vi "OneBallAuton.vi"   [LabVIEW 2013]
uses:
  <vilib>/Rock Robotics/WPI/SafetyOutput/WPI_SafetyOutputConfigMenu.ctl
  <vilib>/Rock Robotics/WPI/Solenoid/WPI_SolenoidValue.ctl
  <vilib>/Rock Robotics/WPI/RobotDrive/WPI_RobotDriveGetSetRefNum.vi
  <vilib>/Rock Robotics/WPI/Solenoid/WPI_SolenoidSetEnum.vi
types:
  T1 = typedef "WPI_SafetyOutputConfigMenu.ctl" = enum16{"Enable", "Disable"}
  T2 = typedef "WPI_RobotDriveDevRef.ctl" = cluster{"DevStatus":errorcluster, "Motors[]":T3[], "Square Inputs":bool, "Max Output":dbl, "Isochronous":bool}
  T3 = typedef "WPI_MotorControlDeviceRef.ctl" = cluster{"DeviceStatus":errorcluster, "Type":enum16{"PWM", "CAN"}, "PWM":cluster{"Digital Module":T4, "PWM Channel":T5, "DeadBand":T6}, "CAN":cluster{"Device Number":u8, "Control Mode":T7, "Semaphore":T8, "Max Vout":dbl}, "Invert":bool, "TransformRef":T9, "InvTransformRef":T9}
  T4 = typedef "FPGA_TypedefDigitalModule.ctl" = enum16{"Digital Module 1", "Digital Module 2"}
  T5 = typedef "FPGA_DIOPWMChannel.ctl" = enum8{"PWM 1", "PWM 2", "PWM 3", "PWM 4", "PWM 5", "PWM 6", "PWM 7", "PWM 8", "PWM 9", "PWM 10", "Invalid"}
  T6 = typedef "WPI_PWMDeadband.ctl" = cluster{"Name":string, "maxPositivePwm":i32, "minPositivePwm":i32, "centerPwm":i32, "maxNegativePwm":i32, "minNegativePwm":i32, "angularRange":u16}
  T7 = typedef "WPI_CANJaguar_ControlMode.ctl" = enum8{"Percent VBus", "Current", "Speed", "Position", "Voltage"}
  T8 = typedef "Semaphore RefNum" = refnum<k1>
  T9 = typedef "WPI_PWMTransform_ConPane.ctl" = refnum<vi>
  T10 = typedef "WPI_SolenoidDevRef.ctl" = cluster{"DevStatus":errorcluster, "Solenoid Module":T11, "Forward Solenoid Channel":T12, "Reverse Solenoid Channel":T12}
  T11 = typedef "FPGA_TypedefSolenoidModule.ctl" = enum16{"Solenoid Module 1", "Solenoid Module 2"}
  T12 = typedef "WPI_SolenoidChannel.ctl" = enum8{"Solenoid 1", "Solenoid 2", "Solenoid 3", "Solenoid 4", "Solenoid 5", "Solenoid 6", "Solenoid 7", "Solenoid 8", "Invalid"}
  T13 = typedef "WPI_DigitalInputDevRef.ctl" = cluster{"DevStatus":errorcluster, "DIO Channel":T14, "Digital Module":T4}
  T14 = typedef "FPGA_DIOChannel.ctl" = enum8{"DIO 1", "DIO 2", "DIO 3", "DIO 4", "DIO 5", "DIO 6", "DIO 7", "DIO 8", "DIO 9", "DIO 10", "DIO 11", "DIO 12", "DIO 13", "DIO 14", "Invalid"}
  T15 = typedef "WPI_EncoderDevRef.ctl" = cluster{"DevStatus":errorcluster, "EncoderIndex":T16, "CounterIndex":T17, "DistancePerCount":dbl, "Decoding Type":T18}
  T16 = typedef "FPGA_EncoderIdx.ctl" = enum8{"Enc 0", "Enc 1", "Enc 2", "Enc 3", "Invalid"}
  T17 = typedef "FPGA_CounterCtrSystemIndex.ctl" = enum8{"Ctr 0", "Ctr 1", "Ctr 2", "Ctr 3", "Ctr 4", "Ctr 5", "Ctr 6", "Ctr 7", "Invalid"}
  T18 = typedef "WPI_EncoderType.ctl" = enum16{"1x", "2x", "4x"}
  T19 = typedef "WPI_SolenoidValue.ctl" = enum16{"Off", "On", "Forward", "Reverse"}
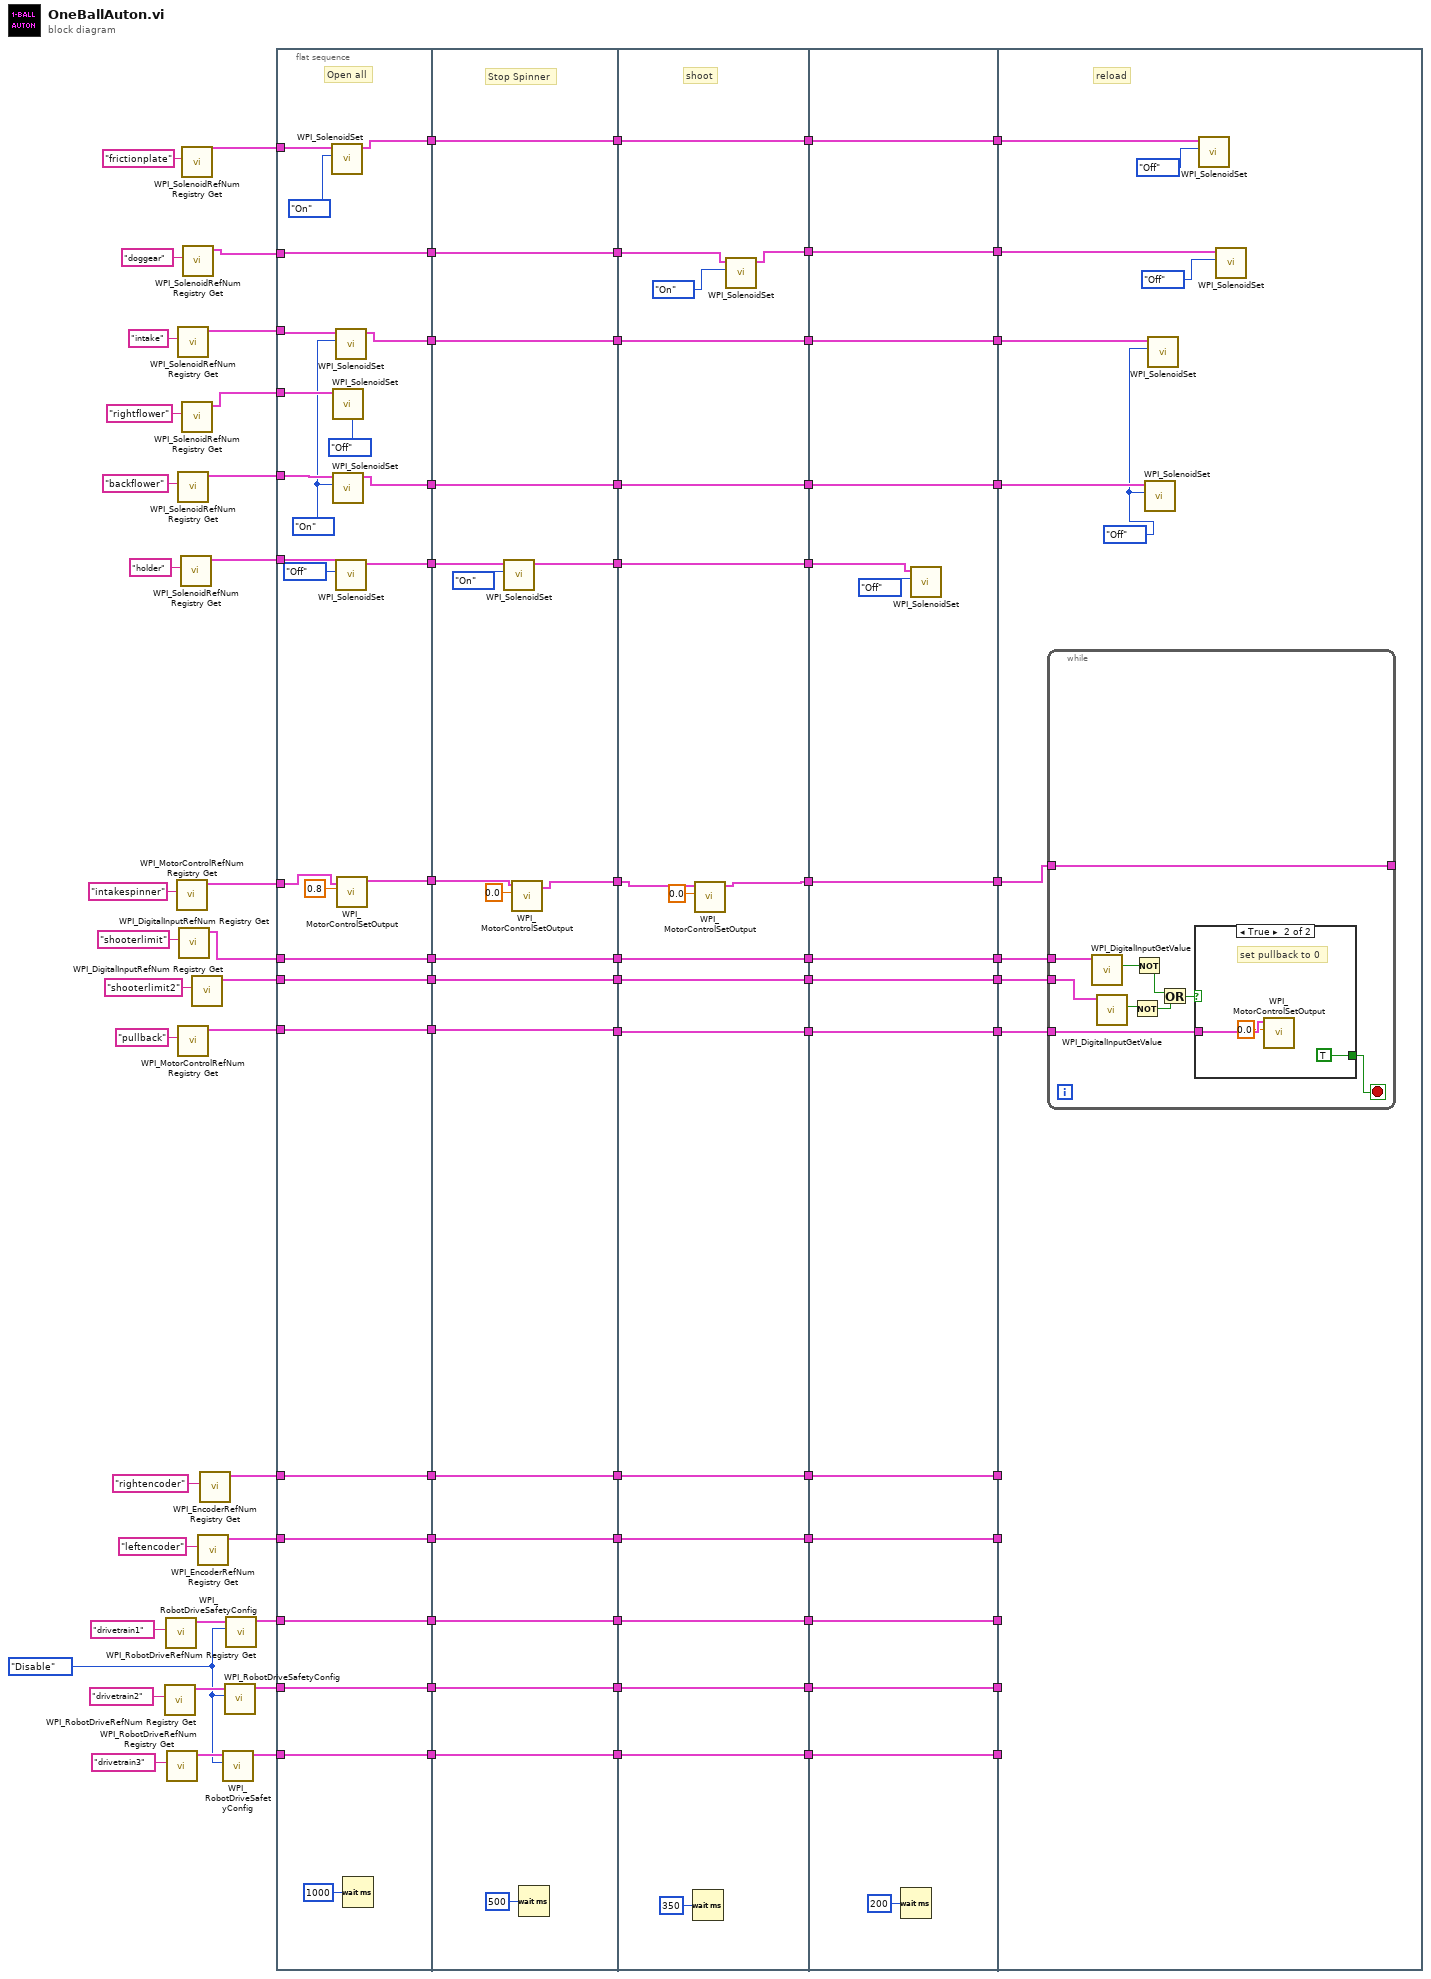
[diagram p0: block diagram]
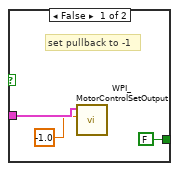
[diagram p2: hidden frame]
diagram:
  w49 = WPI_SafetyOutputConfigMenu."Disable" ("mode")
  n1 = call <vilib>:"WPI_RobotDriveRefNum Registry Get.vi"("refnum name"="drivetrain2") -> ("RobotDriveDevRef"=w51:T2)  [unwired: 9 in, 1 out]
  n2 = call <vilib>:"WPI_RobotDriveRefNum Registry Get.vi"("refnum name"="drivetrain1") -> ("RobotDriveDevRef"=w52:T2)  [unwired: 9 in, 1 out]
  n3 = call <vilib>:"WPI_RobotDriveRefNum Registry Get.vi"("refnum name"="drivetrain3") -> ("RobotDriveDevRef"=w50:T2)  [unwired: 9 in, 1 out]
  n4 = call <vilib>:"WPI_MotorControlRefNum Registry Get.vi"("refnum name"="intakespinner") -> ("MotorControlDevRef"=w62:T3)  [unwired: 9 in, 1 out]
  n5 = call <vilib>:"WPI_SolenoidRefNum Registry Get.vi"("refnum name"="intake") -> ("SolenoidDevRef"=w66:T10)  [unwired: 9 in, 1 out]
  n6 = call <vilib>:"WPI_SolenoidRefNum Registry Get.vi"("refnum name"="backflower") -> ("SolenoidDevRef"=w64:T10)  [unwired: 9 in, 1 out]
  n7 = call <vilib>:"WPI_MotorControlRefNum Registry Get.vi"("refnum name"="pullback") -> ("MotorControlDevRef"=w58:T3)  [unwired: 9 in, 1 out]
  n8 = call <vilib>:"WPI_DigitalInputRefNum Registry Get.vi"("refnum name"="shooterlimit") -> ("DigitalInputDevRef"=w60:T13)  [unwired: 9 in, 1 out]
  n9 = call <vilib>:"WPI_SolenoidRefNum Registry Get.vi"("refnum name"="holder") -> ("SolenoidDevRef"=w30:T10)  [unwired: 9 in, 1 out]
  n10 = call <vilib>:"WPI_SolenoidRefNum Registry Get.vi"("refnum name"="frictionplate") -> ("SolenoidDevRef"=w42:T10)  [unwired: 9 in, 1 out]
  n11 = call <vilib>:"WPI_SolenoidRefNum Registry Get.vi"("refnum name"="rightflower") -> ("SolenoidDevRef"=w65:T10)  [unwired: 9 in, 1 out]
  n12 = call <vilib>:"WPI_SolenoidRefNum Registry Get.vi"("refnum name"="doggear") -> ("SolenoidDevRef"=w70:T10)  [unwired: 9 in, 1 out]
  n13 = call <vilib>:"WPI_DigitalInputRefNum Registry Get.vi"("refnum name"="shooterlimit2") -> ("DigitalInputDevRef"=w34:T13)  [unwired: 9 in, 1 out]
  n14 = call <vilib>:"WPI_EncoderRefNum Registry Get.vi"("refnum name"="leftencoder") -> ("EncoderDevRef"=w47:T15)  [unwired: 9 in, 1 out]
  n15 = call <vilib>:"WPI_EncoderRefNum Registry Get.vi"("refnum name"="rightencoder") -> ("EncoderDevRef"=w48:T15)  [unwired: 9 in, 1 out]
  n16 = call <vilib>:"WPI_RobotDriveSafetyConfig.vi"("mode"=w49, "RobotDriveDevRef"=w50) -> ("RobotDriveDevRef"=w44:T2)  [unwired: 8 in, 1 out]
  n17 = call <vilib>:"WPI_RobotDriveSafetyConfig.vi"("mode"=w49, "RobotDriveDevRef"=w51) -> ("RobotDriveDevRef"=w45:T2)  [unwired: 8 in, 1 out]
  n18 = call <vilib>:"WPI_RobotDriveSafetyConfig.vi"("mode"=w49, "RobotDriveDevRef"=w52) -> ("RobotDriveDevRef"=w46:T2)  [unwired: 8 in, 1 out]
  n19 = flat-sequence {
    tunnel: w70 -> [w115]
    tunnel: [w115] -> w89
    tunnel: w66 -> [w114]
    tunnel: w65 -> [w113]
    tunnel: w64 -> [w112]
    tunnel: w62 -> [w110]
    tunnel: [w108] -> w88
    tunnel: w60 -> [w107]
    tunnel: [w107] -> w87
    tunnel: w58 -> [w106]
    tunnel: [w106] -> w86
    tunnel: [w105] -> w85
    tunnel: w48 -> [w105]
    tunnel: [w104] -> w84
    tunnel: w47 -> [w104]
    tunnel: [w103] -> w83
    tunnel: w46 -> [w103]
    tunnel: [w102] -> w82
    tunnel: w45 -> [w102]
    tunnel: [w101] -> w81
    tunnel: w44 -> [w101]
    tunnel: w42 -> [w98]
    tunnel: [w96] -> w41
    tunnel: [w95] -> w38
    tunnel: [w94] -> w36
    tunnel: w34 -> [w93]
    tunnel: [w93] -> w33
    tunnel: w30 -> [w92]
    tunnel: [w90] -> w29
    tunnel: w89 -> [w128]
    tunnel: w88 -> [w134]
    tunnel: [w131] -> w80
    tunnel: [w130] -> w79
    tunnel: w87 -> [w130]
    tunnel: w86 -> [w129]
    tunnel: [w129] -> w78
    tunnel: [w128] -> w77
    tunnel: w85 -> [w126]
    tunnel: w84 -> [w127]
    tunnel: [w127] -> w76
    tunnel: [w126] -> w75
    tunnel: w83 -> [w125]
    tunnel: w82 -> [w124]
    tunnel: [w125] -> w74
    tunnel: [w124] -> w73
    tunnel: w81 -> [w123]
    tunnel: [w123] -> w72
    tunnel: w41 -> [w122]
    tunnel: [w122] -> w40
    tunnel: [w121] -> w39
    tunnel: w38 -> [w121]
    tunnel: [w120] -> w37
    tunnel: w36 -> [w120]
    tunnel: w33 -> [w119]
    tunnel: [w119] -> w32
    tunnel: w29 -> [w118]
    tunnel: [w116] -> w2
    tunnel: w80 -> [w151]
    tunnel: [w150] -> w12
    tunnel: w79 -> [w153]
    tunnel: [w153] -> w14
    tunnel: w78 -> [w152]
    tunnel: [w152] -> w16
    tunnel: [w146] -> w18
    tunnel: w77 -> [w145]
    tunnel: [w144] -> w20
    tunnel: w76 -> [w144]
    tunnel: [w143] -> w22
    tunnel: w75 -> [w143]
    tunnel: [w142] -> w24
    tunnel: w74 -> [w142]
    tunnel: [w141] -> w26
    tunnel: w73 -> [w141]
    tunnel: [w140] -> w28
    tunnel: w72 -> [w140]
    tunnel: w40 -> [w139]
    tunnel: [w139] -> w10
    tunnel: [w138] -> w8
    tunnel: w39 -> [w138]
    tunnel: [w137] -> w6
    tunnel: w37 -> [w137]
    tunnel: w32 -> [w136]
    tunnel: [w136] -> w4
    tunnel: w2 -> [w135]
    tunnel: [w135] -> w1
    tunnel: w28 -> [w169]
    tunnel: [w169] -> w27
    tunnel: w26 -> [w168]
    tunnel: [w168] -> w25
    tunnel: w24 -> [w167]
    tunnel: [w167] -> w23
    tunnel: w22 -> [w166]
    tunnel: [w166] -> w21
    tunnel: w20 -> [w165]
    tunnel: [w165] -> w19
    tunnel: w18 -> [w164]
    tunnel: [w164] -> w17
    tunnel: w16 -> [w163]
    tunnel: [w163] -> w15
    tunnel: w14 -> [w162]
    tunnel: [w162] -> w13
    tunnel: w12 -> [w161]
    tunnel: [w161] -> w11
    tunnel: w10 -> [w160]
    tunnel: [w160] -> w9
    tunnel: w8 -> [w159]
    tunnel: [w159] -> w7
    tunnel: w6 -> [w158]
    tunnel: [w158] -> w5
    tunnel: w4 -> [w157]
    tunnel: [w157] -> w3
    tunnel: w1 -> [w155]
    tunnel: w27 -> [_]
    tunnel: w25 -> [_]
    tunnel: w23 -> [_]
    tunnel: w21 -> [_]
    tunnel: w19 -> [_]
    tunnel: w17 -> [w176]
    tunnel: w15 -> [w179]
    tunnel: w13 -> [w180]
    tunnel: w11 -> [w178]
    tunnel: w9 -> [w174]
    tunnel: w7 -> [w173]
    tunnel: w5 -> [w172]
    tunnel: w3 -> [w170]
    frame #0 {
      w100 = WPI_SolenoidValue."On" ("Value")
      # "Open all"
      n20 = call-poly <vilib>:"WPI_SolenoidSet.vi"("Value"=WPI_SolenoidValue."On", "SolenoidDevRef"=w98) -> ("SolenoidDevRef"=w96:T10)  [unwired: 8 in, 1 out]
      n21 = call-poly <vilib>:"WPI_SolenoidSet.vi"("Value"=WPI_SolenoidValue."Off", "SolenoidDevRef"=w113) -> ()  [unwired: 8 in, 2 out]
      n22 = call-poly <vilib>:"WPI_SolenoidSet.vi"("Value"=w100, "SolenoidDevRef"=w112) -> ("SolenoidDevRef"=w94:T10)  [unwired: 8 in, 1 out]
      n23 = call-poly <vilib>:"WPI_SolenoidSet.vi"("Value"=w100, "SolenoidDevRef"=w114) -> ("SolenoidDevRef"=w95:T10)  [unwired: 8 in, 1 out]
      n24 = call-poly <vilib>:"WPI_SolenoidSet.vi"("Value"=WPI_SolenoidValue."Off", "SolenoidDevRef"=w92) -> ("SolenoidDevRef"=w90:T10)  [unwired: 8 in, 1 out]
      n25 = call <vilib>:"WPI_MotorControlSetOutput.vi"("Output"=0.8, "MotorControlDevRef"=w110) -> ("MotorControlDevRef"=w108:T3)  [unwired: 7 in, 2 out]
      n26 = Wait (ms)(milliseconds to wait=u32 1000) -> ()  [unwired: 1 out]
    }
    frame #1 {
      # "Stop Spinner"
      n27 = call-poly <vilib>:"WPI_SolenoidSet.vi"("Value"=WPI_SolenoidValue."On", "SolenoidDevRef"=w118) -> ("SolenoidDevRef"=w116:T10)  [unwired: 8 in, 1 out]
      n28 = call <vilib>:"WPI_MotorControlSetOutput.vi"("Output"=0.0, "MotorControlDevRef"=w134) -> ("MotorControlDevRef"=w131:T3)  [unwired: 7 in, 2 out]
      n29 = Wait (ms)(milliseconds to wait=u32 500) -> ()  [unwired: 1 out]
    }
    frame #2 {
      # "shoot"
      n30 = Wait (ms)(milliseconds to wait=u32 350) -> ()  [unwired: 1 out]
      n31 = call <vilib>:"WPI_MotorControlSetOutput.vi"("Output"=0.0, "MotorControlDevRef"=w151) -> ("MotorControlDevRef"=w150:T3)  [unwired: 7 in, 2 out]
      n32 = call-poly <vilib>:"WPI_SolenoidSet.vi"("Value"=WPI_SolenoidValue."On", "SolenoidDevRef"=w145) -> ("SolenoidDevRef"=w146:T10)  [unwired: 8 in, 1 out]
    }
    frame #3 {
      n33 = Wait (ms)(milliseconds to wait=u32 200) -> ()  [unwired: 1 out]
      n34 = call-poly <vilib>:"WPI_SolenoidSet.vi"("Value"=WPI_SolenoidValue."Off", "SolenoidDevRef"=w155) -> ()  [unwired: 8 in, 2 out]
    }
    frame #4 {
      w171 = WPI_SolenoidValue."Off" ("Value")
      # "reload"
      n35 = while {
        tunnel: w180 -> [w190]
        tunnel: w179 -> [w188]
        tunnel: [w186] -> _
        tunnel: w178 -> [w186]
        tunnel: w170 -> [w185]
        stop <- w187 stop-if-true
        n36 = call <vilib>:"WPI_DigitalInputGetValue.vi"("DigitalInputDevRef"=w190) -> ("Value"=w189:bool)  [unwired: 8 in, 2 out]
        n37 = call <vilib>:"WPI_DigitalInputGetValue.vi"("DigitalInputDevRef"=w185) -> ("Value"=w181:bool)  [unwired: 8 in, 2 out]
        n38 = Not(x=w181) -> (.not. x?=w182:bool)
        n39 = Not(x=w189) -> (.not. x?=w184:bool)
        n40 = Or(x=w184, y=w182) -> (x .or. y?=w183:bool)
        n41 = case shown="True" w183 {
          tunnel: w188 -> [w193 w196]
          tunnel: [FALSE TRUE] -> w187
          frame False {
            # "set pullback to -1"
            n42 = call <vilib>:"WPI_MotorControlSetOutput.vi"("Output"=-1.0, "MotorControlDevRef"=w193) -> ()  [unwired: 7 in, 3 out]
          }
          frame True {
            # "set pullback to 0"
            n43 = call <vilib>:"WPI_MotorControlSetOutput.vi"("Output"=0.0, "MotorControlDevRef"=w196) -> ()  [unwired: 7 in, 3 out]
          }
        }
      }
      n44 = call-poly <vilib>:"WPI_SolenoidSet.vi"("Value"=w171, "SolenoidDevRef"=w172) -> ()  [unwired: 8 in, 2 out]
      n45 = call-poly <vilib>:"WPI_SolenoidSet.vi"("Value"=w171, "SolenoidDevRef"=w173) -> ()  [unwired: 8 in, 2 out]
      n46 = call-poly <vilib>:"WPI_SolenoidSet.vi"("Value"=WPI_SolenoidValue."Off", "SolenoidDevRef"=w174) -> ()  [unwired: 8 in, 2 out]
      n47 = call-poly <vilib>:"WPI_SolenoidSet.vi"("Value"=WPI_SolenoidValue."Off", "SolenoidDevRef"=w176) -> ()  [unwired: 8 in, 2 out]
    }
  }
